vi "middle_201720092.vi"() -> ()   [LabVIEW 2019]
panel:
  in  "Piano":T1
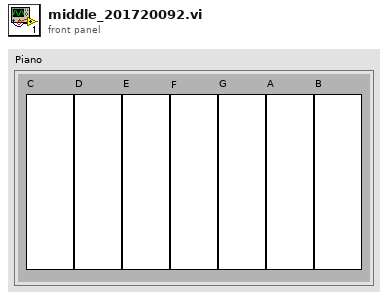
[diagram p1: front panel]
types:
  T1 = cluster{"C":bool, "D":bool, "E":bool, "F":bool, "G":bool, "A":bool, "B":bool}
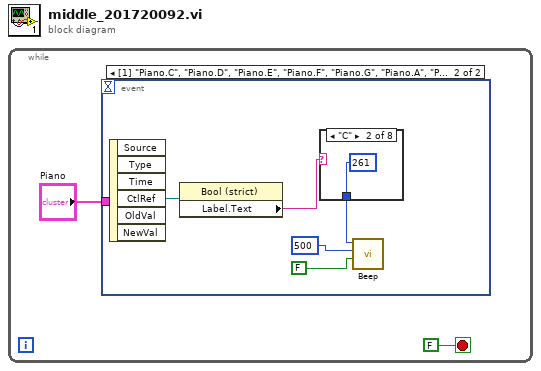
[diagram p0: block diagram]
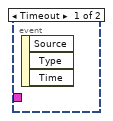
[diagram p2: hidden frame]
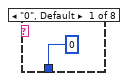
[diagram p3: hidden frame]
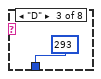
[diagram p4: hidden frame]
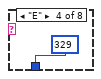
[diagram p5: hidden frame]
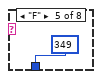
[diagram p6: hidden frame]
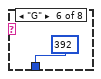
[diagram p7: hidden frame]
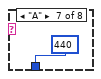
[diagram p8: hidden frame]
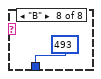
[diagram p9: hidden frame]
diagram:
  n1 = while {
    stop <- FALSE stop-if-true
    n2 = event shown="[1] \"Piano.C\", \"Piano.D\", \"Piano.E\", \"Piano.F\", \"Piano.G\", \"Piano.A\", \"Piano.B\": Value Change" {
      selector: _ -> [_ _]
      dyn-events: _ -> [_ _]
      timeout: _ -> [_ _]
      tunnel: "Piano" -> [_ _]
      event Timeout {
        n3 = event-data() -> ()  [unwired: 1 in, 3 out]
      }
      event "Piano.C", "Piano.D", "Piano.E", "Piano.F", "Piano.G", "Piano.A", "Piano.B": Value Change {
        n4 = event-data() -> ("CtlRef"=w4:refnum<vi>)  [unwired: 1 in, 5 out]
        n5 = property class="Bool (strict)"(reference=w4) -> ("Label.Text"=w3:string)  [unwired: 1 in, 2 out]
        n6 = case shown="\"C\"" w3 {
          tunnel: [u32 0 ("frequency (Hz)") u32 261 ("frequency (Hz)") u32 293 ("frequency (Hz)") u32 329 ("frequency (Hz)") u32 349 ("frequency (Hz)") u32 392 ("frequency (Hz)") u32 440 ("frequency (Hz)") u32 493 ("frequency (Hz)")] -> w5
          frame "0", Default {
          }
          frame "C" {
          }
          frame "D" {
          }
          frame "E" {
          }
          frame "F" {
          }
          frame "G" {
          }
          frame "A" {
          }
          frame "B" {
          }
        }
        n7 = call <vilib>:"Beep.vi"("use system alert? (T)"=FALSE, "duration (msec)"=u32 500, "frequency (Hz)"=w5) -> ()  [unwired: 9 in]
      }
    }
  }
